vi "Determine Y Scale Limits.vi"(8 "error in (no error)":errorcluster, 10 "Volts/Div":string) -> (0 "error out":errorcluster, 1 "Y Min":dbl, 2 "Y Max":dbl, 3 "Volts/Div":dbl, 5 "Units":string)   [LabVIEW 2018]
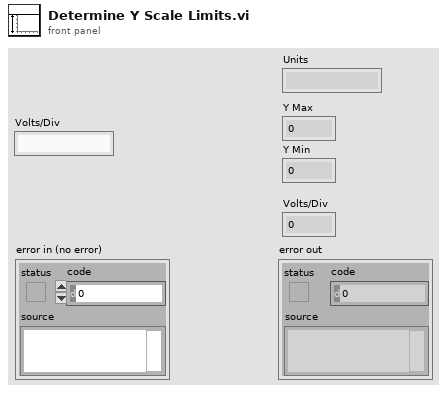
[diagram p1: front panel]
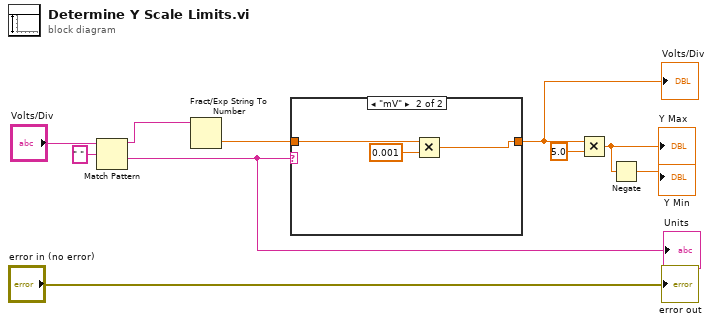
[diagram p0: block diagram]
diagram:
  n1 = Match Pattern(string="Volts/Div", regular expression=" ") -> (before substring=w7:string, after substring=w8:string)  [unwired: 1 in, 2 out]
  "Units" <- w8
  n2 = Fract/Exp String To Number(string=w7) -> (number=w6:dbl)  [unwired: 3 in, 1 out]
  n3 = case shown="\"mV\"" w8 {
    tunnel: w6 -> [w11 w14]
    tunnel: [w11 w12] -> w5
    frame "V", Default {
    }
    frame "mV" {
      n4 = Multiply(x=w14, y=0.001) -> (x*y=w12:dbl)
    }
  }
  "Volts/Div" <- w5
  n5 = Multiply(x=w5, y=5.0) -> (x*y=w3:dbl)
  "Y Max" <- w3
  n6 = Negate(x=w3) -> (-x=→"Y Min":dbl)
  "error out" <- "error in (no error)"
